vi "ReadDecimal.vi"() -> (3 "Флаг Разделителя":bool)   [LabVIEW 2017]
uses:
  <vilib>/registry/registry.llb/Registry RtKey.ctl
  <vilib>/registry/registry.llb/Read Registry Value Simple STR.vi
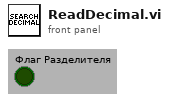
[diagram p1: front panel]
types:
  T1 = typedef "Registry RtKey.ctl" = enum32{"HKEY_CLASSES_ROOT", "HKEY_CURRENT_USER", "HKEY_LOCAL_MACHINE", "HKEY_USERS", "HKEY_PERFORMANCE_DATA", "HKEY_CURRENT_CONFIG", "HKEY_DYN_DATA"}
  T2 = typedef "Registry refnum.ctl" = refnum<k1>
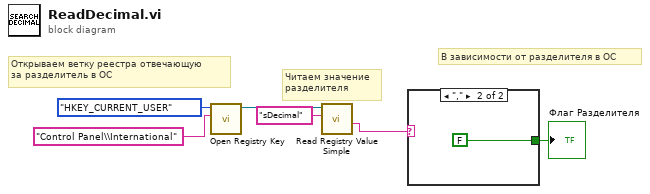
[diagram p0: block diagram]
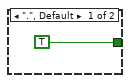
[diagram p2: hidden frame]
diagram:
  # "В зависимости от разделителя в ОС"
  # "Читаем значение\nразделителя"
  # "Открываем ветку реестра отвечающую\nза разделитель в ОС"
  n1 = call <vilib>:"Open Registry Key.vi"("subkey"="Control Panel\\International", "root key (HKEY_LOCAL_MACHINE)"=Registry_RtKey."HKEY_CURRENT_USER") -> ("refnum out"=w5:T2)  [unwired: 8 in, 1 out]
  n2 = call-poly <vilib>:"Read Registry Value Simple.vi"("value"="sDecimal", "refnum"=w5) -> ("String/Binary data"=w2:string)  [unwired: 4 in, 3 out]
  n3 = case shown="\",\"" w2 {
    tunnel: [TRUE FALSE] -> w1
    frame ".", Default {
    }
    frame "," {
    }
  }
  "Флаг Разделителя" <- w1
